vi "Config ACTION.vi"(8 "error in (no error)":errorcluster, 11 "Relev in":refnum<class "Relev.lvclass">) -> (0 "error out":errorcluster, 3 "Relev out":refnum<class "Relev.lvclass">)   [LabVIEW 2014, in "SeqLoop.lvlib" / "STEP Classes.lvlib" / "Relev.lvclass"]
uses:
  Relev.lvclass
  Relev.lvclass/Relev.ctl
panel:
  in  "Relevar Patrón?":bool
  in  "Nº de Transductor para Relevar Patron":i32=1 min=1 format="T%d"
  in  "Cancel":bool
  in  "Save":bool
  # "Dispositivos de Hardware para relevamiento"
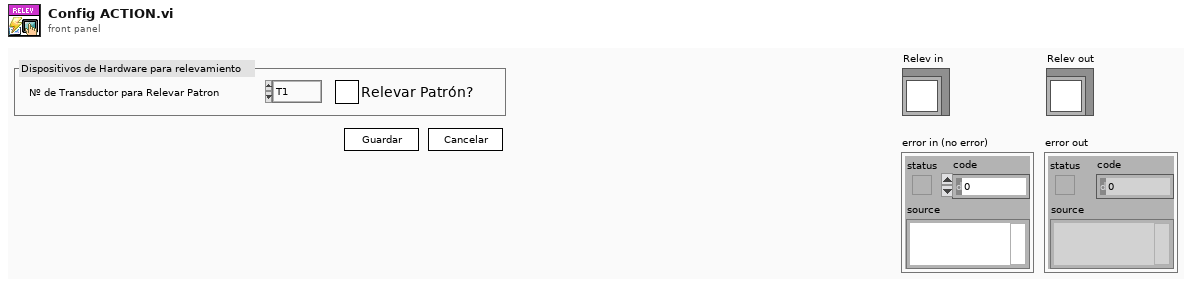
[diagram p1: front panel]
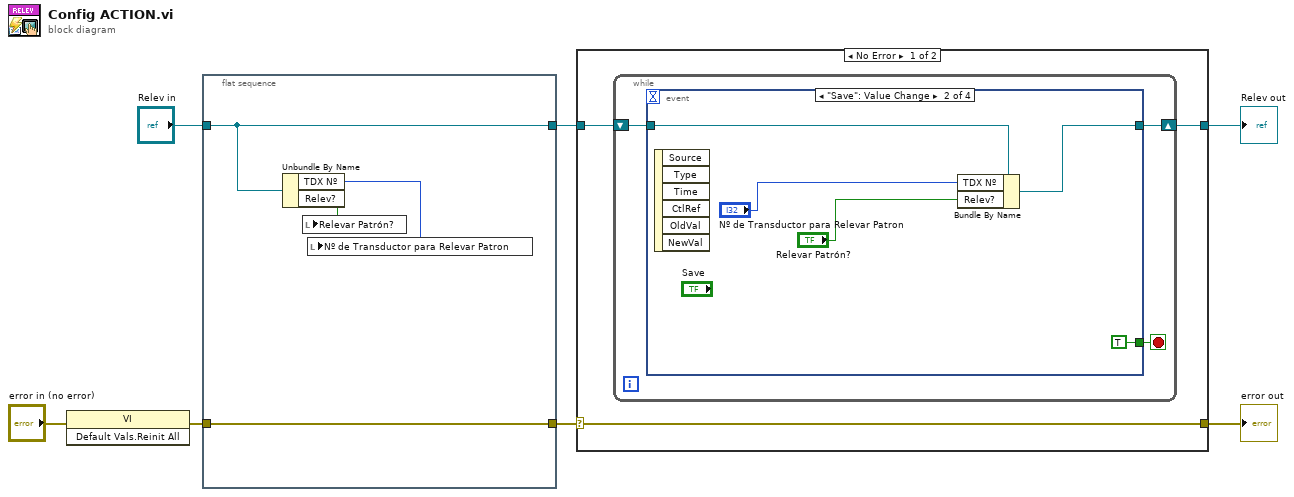
[diagram p0: block diagram]
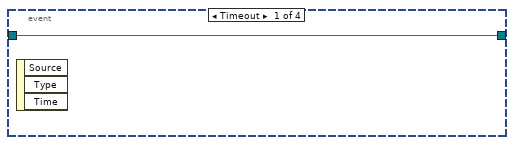
[diagram p2: hidden frame]
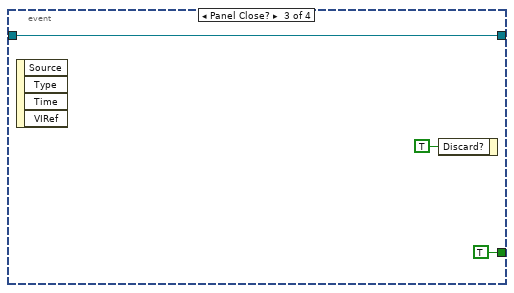
[diagram p3: hidden frame]
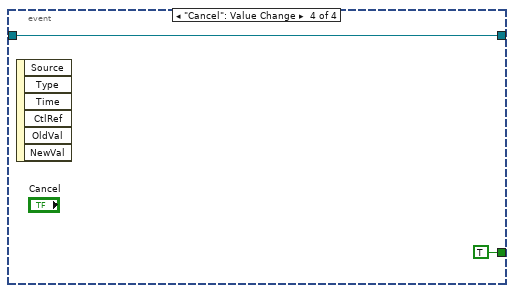
[diagram p4: hidden frame]
diagram:
  n1 = invoke class="VI" method="Default Vals.Reinit All"(error in="error in (no error)") -> (error out=w6:errorcluster)  [unwired: 2 in, 2 out]
  n2 = flat-sequence {
    tunnel: "Relev in" -> [w11]
    tunnel: [w10] -> w7
    tunnel: w6 -> [w10]
    tunnel: [w11] -> w5
    frame #0 {
      n3 = Unbundle By Name(w11) -> ("TDX Nº"=w9:i32, "Relev?"=w8:bool)
      n4 = local write "Relevar Patrón?"(w8) -> ()
      n5 = local write "Nº de Transductor para Relevar Patron"(w9) -> ()
    }
  }
  n6 = case shown="No Error" w7 {
    selector: w7 -> [w14 w30]
    tunnel: [w14 w30] -> w1
    tunnel: [w12 w29] -> w2
    tunnel: w5 -> [w13 w29]
    frame No Error {
      n7 = while {
        shift-right: [w16] -> w12
        shift-left: w13 -> [w17]
        stop <- w15 stop-if-true
        n8 = event shown="[1] \"Save\": Value Change" {
          selector: _ -> [_ _ _ _]
          dyn-events: _ -> [_ _ _ _]
          timeout: _ -> [_ _ _ _]
          tunnel: w17 -> [w18 w22 w26 w28]
          tunnel: [w18 w21 w26 w28] -> w16
          tunnel: [_ TRUE TRUE TRUE] -> w15
          event Timeout {
            n9 = event-data() -> ()  [unwired: 1 in, 3 out]
          }
          event "Save": Value Change {
            n10 = event-data() -> ()  [unwired: 1 in, 6 out]
            n11 = Bundle By Name(cluster=w22, "TDX Nº"="Nº de Transductor para Relevar Patron", "Relev?"="Relevar Patrón?") -> (w21:refnum<class "Relev.lvclass">)
          }
          event Panel Close? {
            n12 = event-data() -> ()  [unwired: 1 in, 4 out]
            n13 = event-data("Discard?"=TRUE) -> ()  [unwired: 1 in, 1 out]
          }
          event "Cancel": Value Change {
            n14 = event-data() -> ()  [unwired: 1 in, 6 out]
          }
        }
      }
    }
    frame Error {
    }
  }
  "error out" <- w1
  "Relev out" <- w2
